vi "AG34980A_Is_Channel_Closed.vi"(0 "VISA resource name":refnum<visa-resource-name>, 1 "Channel List":string, 11 "error in (no error)":errorcluster) -> (4 "VISA resource name out":refnum<visa-resource-name>, 8 "Channel Status (Closed = True)":bool[](array[boolean]), 15 "error out":errorcluster)   [LabVIEW 2022 SP3]
doc: "This VI returns the state (closed = True) of each of the channels specified in the channel list."
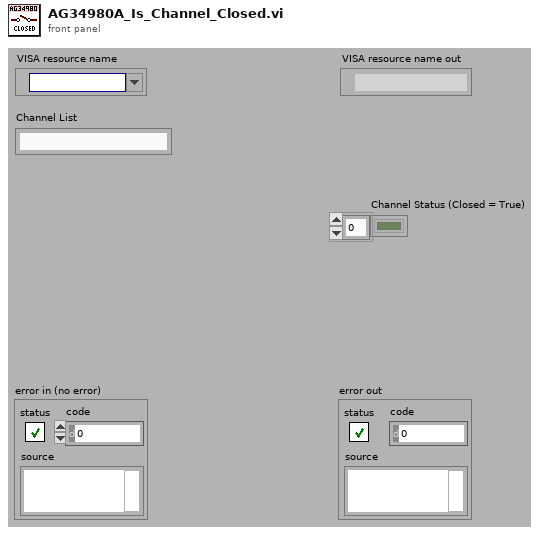
[diagram p1: front panel]
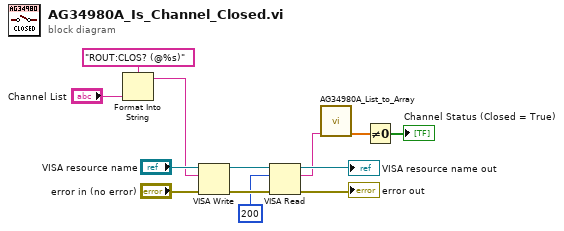
[diagram p0: block diagram]
diagram:
  n1 = Format Into String(format string="ROUT:CLOS? (@%s)", "Channel List") -> (resulting string=w9:string)  [unwired: 2 in, 1 out]
  n2 = VISA Write(VISA resource name="VISA resource name", write buffer=w9, error in (no error)="error in (no error)") -> (VISA resource name out=w8:refnum<visa-resource-name>, error out=w7:errorcluster)  [unwired: 1 out]
  n3 = VISA Read(VISA resource name=w8, byte count=u32 200, error in (no error)=w7) -> (VISA resource name out=→"VISA resource name out":refnum<visa-resource-name>, read buffer=w2:string, error out=→"error out":errorcluster)  [unwired: 1 out]
  n4 = call "AG34980A_List_to_Array.vi"("List"=w2) -> ("Output Number Array"=w1:dbl[])  [unwired: 5 in, 1 out]
  n5 = Not Equal To 0?(x=w1) -> (x != 0?=→"Channel Status (Closed = True)":bool[])
